vi "iter_resetable.vi"(7 "reset":bool) -> (0 "iter":i16)   [LabVIEW 2017, in "libimaging-cs.lvlib"]
doc: "Provides a counter that \nresetts itself ever N iterations.\n\nAt the Nth iteration, the boolean \ntriggers HIGH."
uses:
  libimaging-cs.lvlib
panel:
  # "Provides a counter that \nresetts when reset=True."
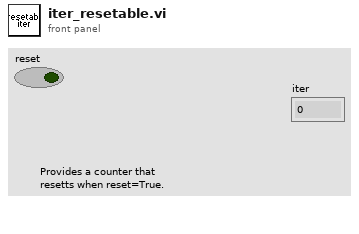
[diagram p1: front panel]
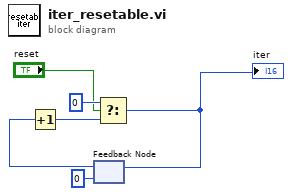
[diagram p0: block diagram]
diagram:
  n1 = feedback #1(i16 0) -> (w5:i16)
  n2 = Increment(x=w5) -> (x+1=w4:i16)
  n3 = Select(t=i16 0, s="reset", f=w4) -> (s? t:f=w1:i16)
  "iter" <- w1
  n4 = feedback-in #1(w1) -> ()
